vi "findCalibrationFactor.vi"() -> ()   [LabVIEW 2015]
uses:
  <vilib>/Analysis/NI_AALPro.lvlib
panel:
  out "Kalibreringsfaktorer":dbl[](array[numeric])
  out "?":string
  out "Punkter":cluster{"Y":dbl[], "Y":dbl[]}[](graph)
  out "Table Control":string[][](table) caption="tabell"
  in  "OK Button 2":bool
  in  "OK Button":bool
  in  "Deformasjon":dbl
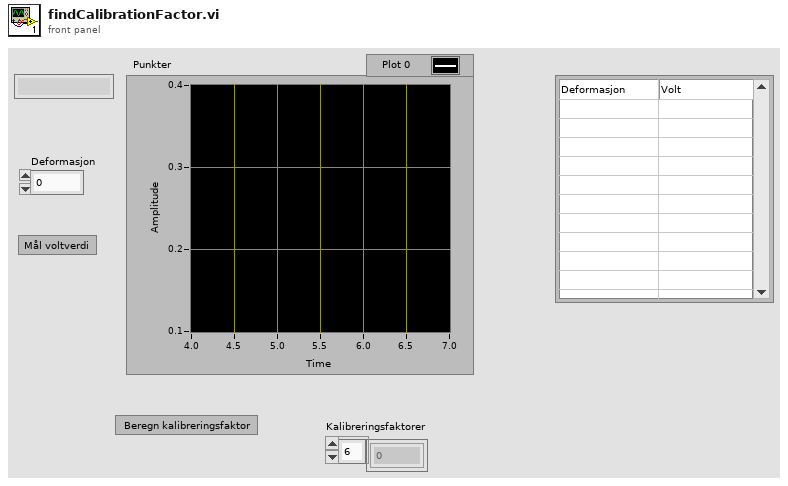
[diagram p1: front panel]
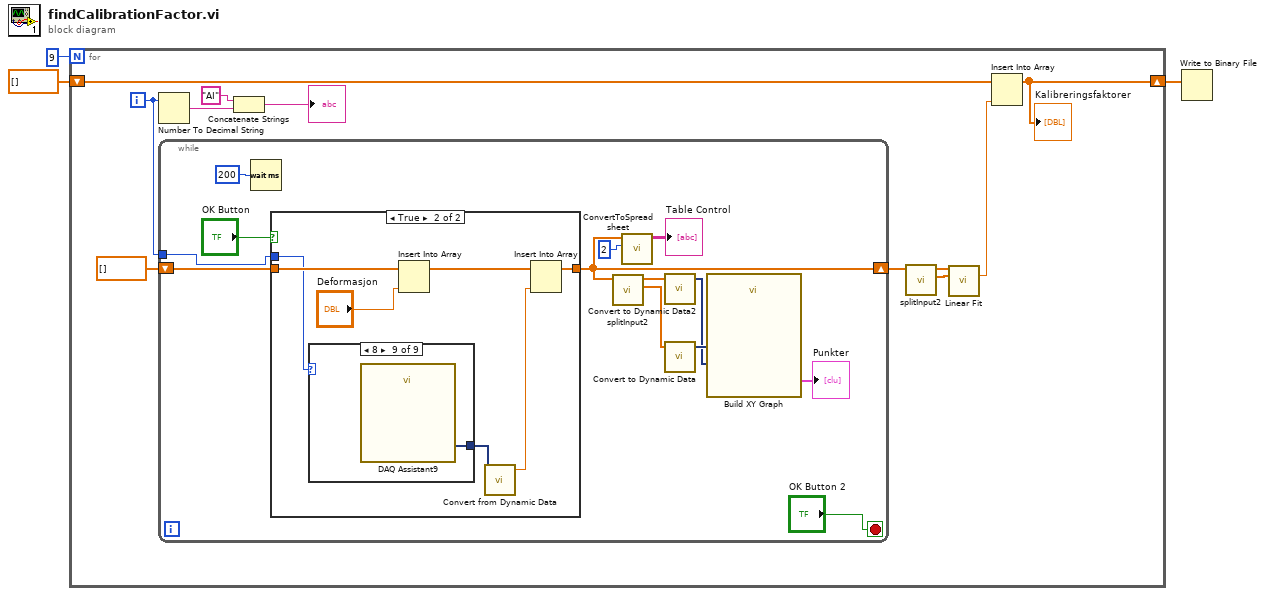
[diagram p0: block diagram]
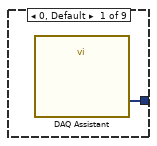
[diagram p3: hidden frame]
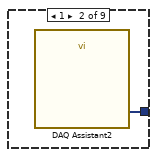
[diagram p4: hidden frame]
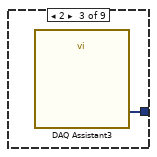
[diagram p5: hidden frame]
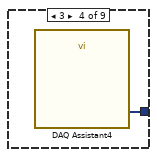
[diagram p6: hidden frame]
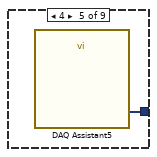
[diagram p7: hidden frame]
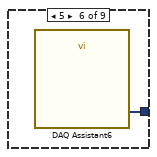
[diagram p8: hidden frame]
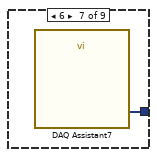
[diagram p9: hidden frame]
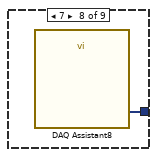
[diagram p10: hidden frame]
diagram:
  n1 = for {
    N: 9 -> [_]
    shift-right: [w5] -> w3
    shift-left: dbl[] [] ("Array") -> [w6]
    i -> [w4]
    n2 = Number To Decimal String(number=w4) -> (decimal integer string=w9:string)  [unwired: 1 in]
    n3 = while {
      shift-right: [w22] -> w13
      shift-left: dbl[] [] ("Array") -> [w25]
      tunnel: w4 -> [w15]
      stop <- "OK Button 2" stop-if-true
      n4 = Wait (ms)(milliseconds to wait=200) -> ()  [unwired: 1 out]
      n5 = case shown="True" "OK Button" {
        tunnel: w25 -> [w28 w35]
        tunnel: [w28 w32] -> w22
        tunnel: w15 -> [_ w29]
        frame False {
        }
        frame True {
          n6 = case shown="8" w29 {
            tunnel: [w36 w37 w38 w39 w40 w41 w42 w43 w44] -> w30
            frame 0, Default {
              n7 = call "DAQ Assistant"() -> ("data"=w36:dynamicdata)  [unwired: 17 in, 2 out]
            }
            frame 1 {
              n8 = call "DAQ Assistant2"() -> ("data"=w37:dynamicdata)  [unwired: 17 in, 2 out]
            }
            frame 2 {
              n9 = call "DAQ Assistant3"() -> ("data"=w38:dynamicdata)  [unwired: 17 in, 2 out]
            }
            frame 3 {
              n10 = call "DAQ Assistant4"() -> ("data"=w39:dynamicdata)  [unwired: 17 in, 2 out]
            }
            frame 4 {
              n11 = call "DAQ Assistant5"() -> ("data"=w40:dynamicdata)  [unwired: 17 in, 2 out]
            }
            frame 5 {
              n12 = call "DAQ Assistant6"() -> ("data"=w41:dynamicdata)  [unwired: 17 in, 2 out]
            }
            frame 6 {
              n13 = call "DAQ Assistant7"() -> ("data"=w42:dynamicdata)  [unwired: 17 in, 2 out]
            }
            frame 7 {
              n14 = call "DAQ Assistant8"() -> ("data"=w43:dynamicdata)  [unwired: 17 in, 2 out]
            }
            frame 8 {
              n15 = call "DAQ Assistant9"() -> ("data"=w44:dynamicdata)  [unwired: 17 in, 2 out]
            }
          }
          n16 = Insert Into Array(array=w35, new element="Deformasjon") -> (w33:dbl[])  [unwired: 1 in]
          n17 = call "Convert from Dynamic Data"("Dynamic Data Type"=w30) -> ("Scalar"=w31:dbl)  [unwired: 3 in]
          n18 = Insert Into Array(array=w33, new element=w31) -> (w32:dbl[])  [unwired: 1 in]
        }
      }
      n19 = call "splitInput2.vi"("Array"=w22) -> ("Defromasjon"=w20:dbl[], "Volt"=w18:dbl[])  [unwired: 9 in]
      n20 = call "ConvertToSpreadsheet.vi"("Kolonner"=2, "Array in"=w22) -> ("Array out"=→"Table Control":string[][])  [unwired: 9 in]
      n21 = call "Convert to Dynamic Data2"("Array"=w18) -> ("Dynamic Data Type"=w17:dynamicdata)  [unwired: 3 in]
      n22 = call "Convert to Dynamic Data"("Array"=w20) -> ("Dynamic Data Type"=w19:dynamicdata)  [unwired: 3 in]
      n23 = call "Build XY Graph"("Y Input"=w17, "X Input"=w19) -> ("XY Graph"=→"Punkter":cluster{"X":dbl[], "Y":dbl[]}[])  [unwired: 8 in, 1 out]
    }
    n24 = Concatenate Strings("AI", w9) -> (→"?":string)
    n25 = call "splitInput2.vi"("Array"=w13) -> ("Defromasjon"=w12:dbl[], "Volt"=w11:dbl[])  [unwired: 9 in]
    n26 = call <vilib>:"Linear Fit.vi"("Y"=w11, "X"=w12) -> ("slope"=w7:dbl)  [unwired: 9 in, 4 out]
    n27 = Insert Into Array(array=w6, new element=w7) -> (w5:dbl[])  [unwired: 1 in]
    "Kalibreringsfaktorer" <- w5
  }
  n28 = Write to Binary File(data=w3) -> ()  [unwired: 5 in, 3 out]
